vi "myRIOminiVoiceCommand.vi"() -> ()   [LabVIEW 2019]
uses:
  VoiceCommandState.ctl
  <vilib>/myRIO/Common/Instrument Driver Framework/myRIO v1.0/UART/vis/myRIO v1.0 Close UART.vi
  <vilib>/myRIO/Common/Instrument Driver Framework/Utilities/vis/FPGA Ref Manager.vi
  <vilib>/myRIO/Common/Instrument Driver Framework/myRIO v1.0/myRIO v1.0 Reset FPGA.vi
  <vilib>/myRIO/Common/Instrument Driver Framework/myRIO v1.0/IRQ/vis/myRIO v1.0 IRQ Info FGV.vi
  <vilib>/myRIO/Common/Instrument Driver Framework/myRIO v1.0/IRQ/vis/myRIO v1.0 Timer IRQ Info FGV.vi
  <vilib>/myRIO/Common/Instrument Driver Framework/myRIO v1.0/IRQ/vis/myRIO v1.0 ISR Agent.vi
  <vilib>/myRIO/Instrument Drivers/Utilities/vis/Reset Index.vi
  <vilib>/myRIO/Common/Instrument Driver Framework/myRIO v1.0/Resource Manager/vis/myRIO v1.0 Block Write Resource Manager.vi
  Simple Queue Message/Simple Queue Message.lvlib
  <vilib>/myRIO/Instrument Drivers/Utilities/Utilities.lvlib
  Downloads/DFRobot_ASR_myRIO_Lib_ProgramProject/DFRROBOT_ASR_myRIO_Lib/DFRobot_ASR_myRIO.lvlib
panel:
  out "Result out":i32
  out "output array":dbl[][](array[numeric])
  out "heard":i32
  out "distance":i32
  out "command":i32
  out "Correct Key?":bool
  out "Battery (Volts)":dbl format="%.1f"
  out "State":T1
  in  "Stop Button":bool
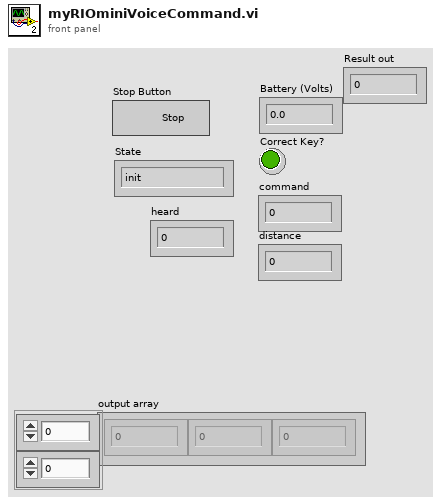
[diagram p1: front panel]
types:
  T1 = typedef "VoiceCommandState.ctl" = enum16{"init", "command", "quantity", "finish", "err"}
  T2 = typedef "miniRef.ctl" = cluster{"Custom FPGA Reference":refnum<k20>, "error out":errorcluster}
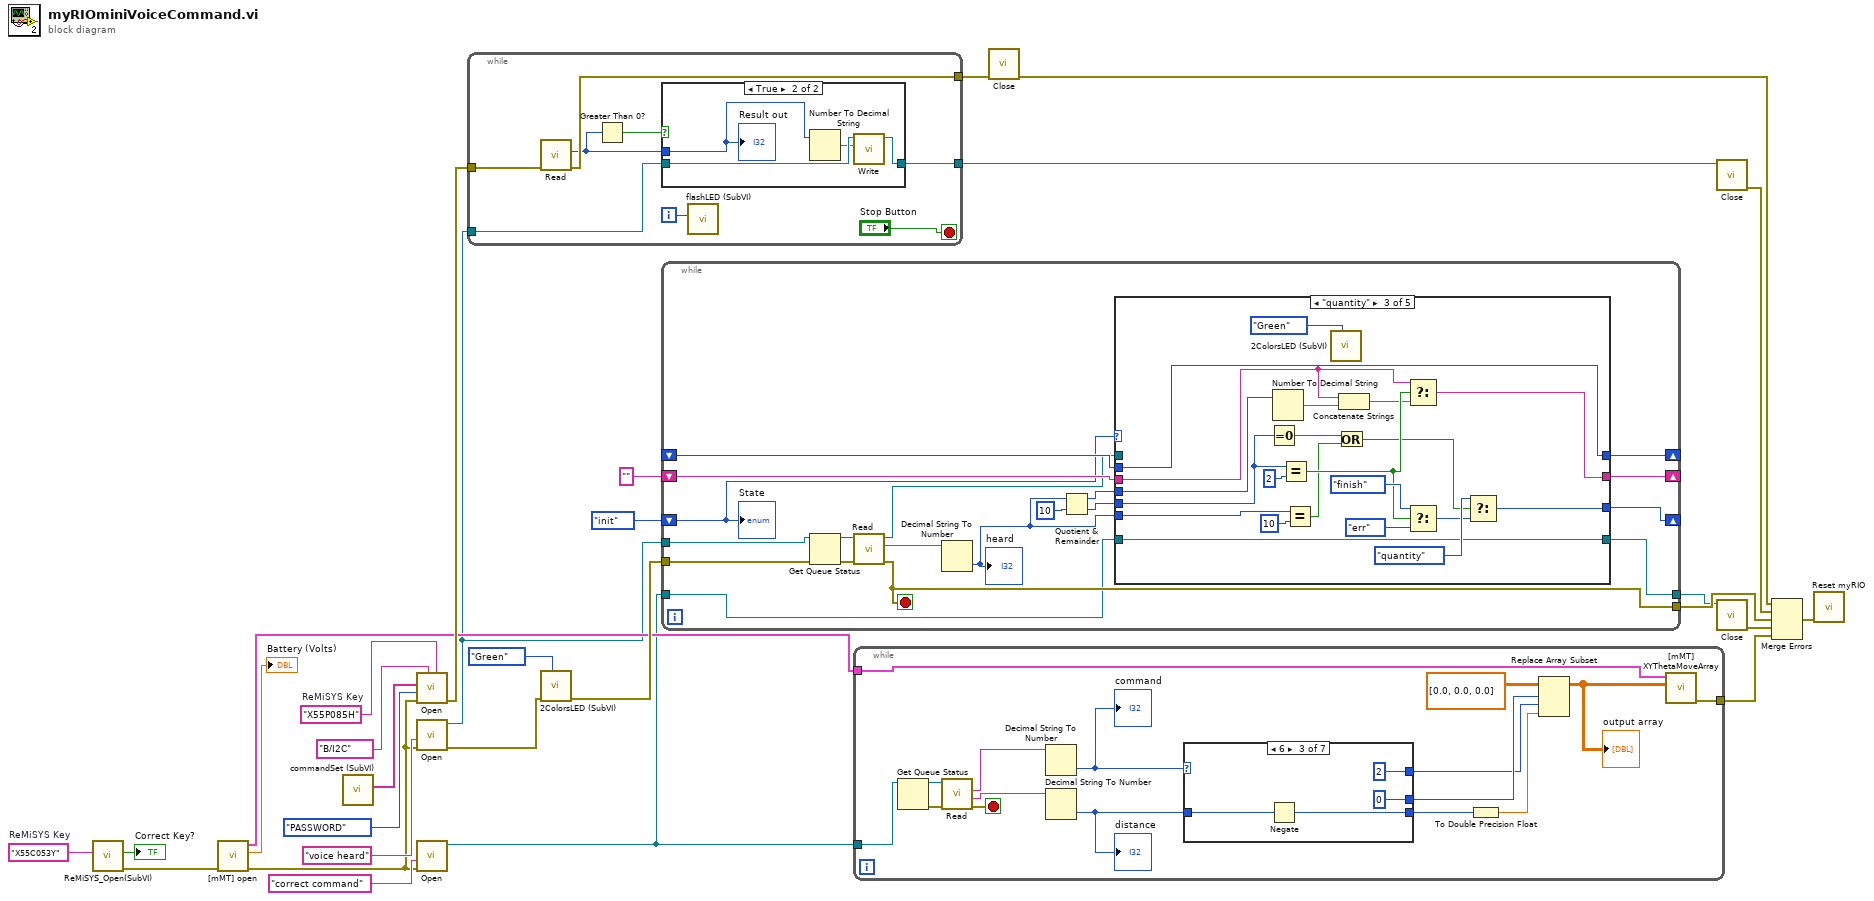
[diagram p0: block diagram]
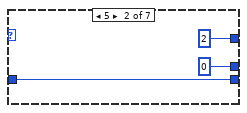
[diagram p3: hidden frame]
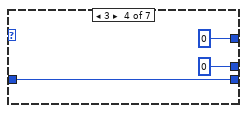
[diagram p4: hidden frame]
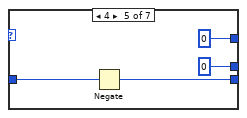
[diagram p5: hidden frame]
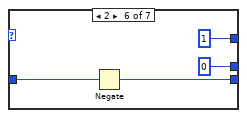
[diagram p6: hidden frame]
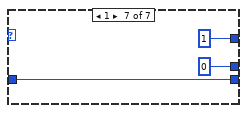
[diagram p7: hidden frame]
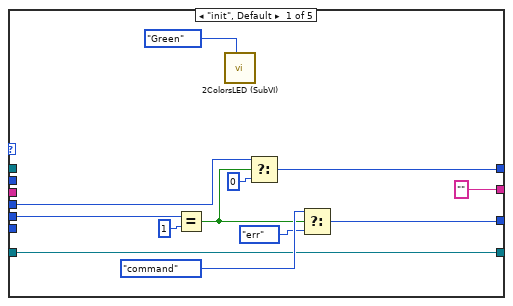
[diagram p8: hidden frame]
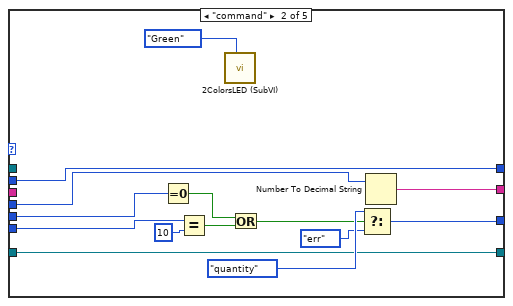
[diagram p9: hidden frame]
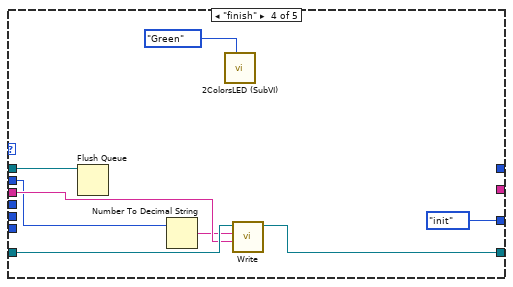
[diagram p10: hidden frame]
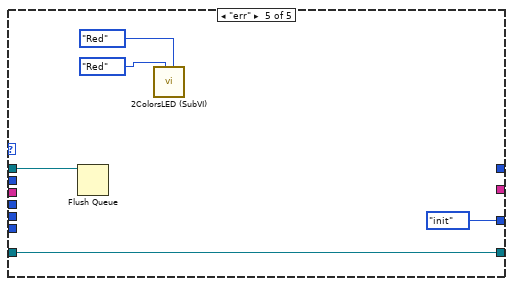
[diagram p11: hidden frame]
diagram:
  w9 = "X55C053Y"  # ReMiSYS Key
  w29 = "X55P085H"  # ReMiSYS Key
  n1 = call <vilib>:"ReMiSYS_Open(SubVI).vi"("ReMiSYS Key"=w9) -> ("error out"=w8:errorcluster, "Correct Key?"=→"Correct Key?":bool)  [unwired: 9 in]
  n2 = call <vilib>:"[mMT] open.vi"("error in"=w8) -> ("error out"=w1:errorcluster, "Battery (Volts)"=→"Battery (Volts)":dbl, "miniOut"=w7:T2)  [unwired: 8 in]
  n3 = call "commandSet (SubVI).vi"() -> ("CommandSet"=w19:string[])  [unwired: 11 in]
  n4 = call "Open.vi"("ReMiSYS Key"=w29, "Channel Name"=tag "B/I2C", "error in (no error)"=w1, "eMode"=enum16{"LOOP", "PASSWORD", "BUTTON"}."PASSWORD", "Command"=w19) -> ("error out"=w28:errorcluster)  [unwired: 6 in]
  n5 = call "Open.vi"("error in (no error)"=w1, "name (unnamed)"="voice heard") -> ("error out"=w15:errorcluster, "queue out"=w2:refnum<queue>)  [unwired: 8 in]
  n6 = call "Open.vi"("error in (no error)"=w1, "name (unnamed)"="correct command") -> ("queue out"=w3:refnum<queue>)  [unwired: 8 in, 1 out]
  n7 = while {
    tunnel: w28 -> [w37]
    tunnel: [w36] -> w25
    tunnel: w2 -> [w34]
    tunnel: [w33] -> w23
    i -> [w30]
    stop <- "Stop Button" stop-if-true
    n8 = call "Read.vi"("error in (no error)"=w37) -> ("error out"=w36:errorcluster, "Result out"=w32:i32)  [unwired: 9 in]
    n9 = Greater Than 0?(x=w32) -> (x > 0?=w31:bool)
    n10 = case shown="True" w31 {
      tunnel: w34 -> [w38 w42]
      tunnel: [w38 w41] -> w33
      tunnel: w32 -> [_ w40]
      frame False {
      }
      frame True {
        n11 = Number To Decimal String(number=w40) -> (decimal integer string=w39:string)  [unwired: 1 in]
        n12 = call "Write.vi"("state"=w39, "queue"=w42) -> ("queue out"=w41:refnum<queue>)  [unwired: 8 in, 1 out]
        "Result out" <- w40
      }
    }
    n13 = call "flashLED (SubVI).vi"("i"=w30) -> ()  [unwired: 11 in]
  }
  n14 = call "2ColorsLED (SubVI).vi"("Color"=enum16{"Green", "Red", "Dimm"}."Green", "error in (no error)"=w15) -> ("error out"=w14:errorcluster)  [unwired: 9 in]
  n15 = while {
    tunnel: w2 -> [w51]
    shift-right: [w60] -> _
    shift-left: VoiceCommandState."init" -> [w47]
    shift-right: [w57] -> _
    shift-left: "" -> [w56]
    shift-right: [w54] -> _
    shift-left: _ -> [w53]
    tunnel: [w48] -> w16
    tunnel: w14 -> [w45]
    tunnel: w3 -> [w44]
    tunnel: [w43] -> w11
    stop <- w48 stop-if-true
    n16 = Get Queue Status(queue=w51, error in (no error)=w45) -> (queue out=w50:refnum<queue>, error out=w49:errorcluster)  [unwired: 1 in, 6 out]
    n17 = call "Read.vi"("error in (no error)"=w49, "queue"=w50) -> ("error out"=w48:errorcluster, "state"=w61:string, "queue out"=w52:refnum<queue>)  [unwired: 6 in, 1 out]
    n18 = Decimal String To Number(string=w61) -> (number=w46:i32)  [unwired: 2 in, 1 out]
    "heard" <- w46
    n19 = Quotient & Remainder(x=w46, y=10) -> (x-y*floor(x/y)=w55:i32, floor(x/y)=w58:i32)
    n20 = case shown="\"quantity\"" w47 {
      tunnel: [w70 w87 w100 VoiceCommandState."init" VoiceCommandState."init"] -> w60
      tunnel: w58 -> [w69 w82 w106 _ _]
      tunnel: ["" w84 w96 _ _] -> w57
      tunnel: w56 -> [_ _ w98 w112 _]
      tunnel: [w66 w83 w101 _ _] -> w54
      tunnel: w55 -> [w67 w81 w88 _ _]
      tunnel: w53 -> [_ w83 w101 w109 _]
      tunnel: w52 -> [_ _ _ w115 w121]
      tunnel: w46 -> [_ w79 w90 _ _]
      tunnel: w44 -> [w62 w74 w94 w113 w117]
      tunnel: [w62 w74 w94 w111 w117] -> w43
      frame "init", Default {
        n21 = Equal?(x=w69, y=1) -> (x = y?=w68:bool)
        n22 = call "2ColorsLED (SubVI).vi"("Color"=enum16{"Green", "Red", "Dimm"}."Green") -> ()  [unwired: 10 in, 1 out]
        n23 = Select(t=w67, s=w68, f=0) -> (s? t:f=w66:i32)
        n24 = Select(t=VoiceCommandState."command", s=w68, f=VoiceCommandState."err") -> (s? t:f=w70:T1)
      }
      frame "command" {
        n25 = Equal To 0?(x=w82) -> (x = 0?=w80:bool)
        n26 = Equal?(x=w79, y=10) -> (x = y?=w77:bool)
        n27 = call "2ColorsLED (SubVI).vi"("Color"=enum16{"Green", "Red", "Dimm"}."Green") -> ()  [unwired: 10 in, 1 out]
        n28 = Or(x=w80, y=w77) -> (x .or. y?=w76:bool)
        n29 = Select(t=VoiceCommandState."quantity", s=w76, f=VoiceCommandState."err") -> (s? t:f=w87:T1)
        n30 = Number To Decimal String(number=w81) -> (decimal integer string=w84:string)  [unwired: 1 in]
      }
      frame "quantity" {
        n31 = Equal To 0?(x=w106) -> (x = 0?=w91:bool)
        n32 = Number To Decimal String(number=w88) -> (decimal integer string=w108:string)  [unwired: 1 in]
        n33 = Equal?(x=w106, y=2) -> (x = y?=w99:bool)
        n34 = Equal?(x=w90, y=10) -> (x = y?=w92:bool)
        n35 = call "2ColorsLED (SubVI).vi"("Color"=enum16{"Green", "Red", "Dimm"}."Green") -> ()  [unwired: 10 in, 1 out]
        n36 = Or(x=w91, y=w92) -> (x .or. y?=w89:bool)
        n37 = Concatenate Strings(w98, w108) -> (w97:string)
        n38 = Select(t=w98, s=w99, f=w97) -> (s? t:f=w96:string)
        n39 = Select(t=VoiceCommandState."finish", s=w99, f=VoiceCommandState."err") -> (s? t:f=w103:T1)
        n40 = Select(t=VoiceCommandState."quantity", s=w89, f=w103) -> (s? t:f=w100:T1)
      }
      frame "finish" {
        n41 = Flush Queue(queue=w115) -> ()  [unwired: 1 in, 3 out]
        n42 = Number To Decimal String(number=w109) -> (decimal integer string=w110:string)  [unwired: 1 in]
        n43 = call "2ColorsLED (SubVI).vi"("Color"=enum16{"Green", "Red", "Dimm"}."Green") -> ()  [unwired: 10 in, 1 out]
        n44 = call "Write.vi"("payload"=w112, "state"=w110, "queue"=w113) -> ("queue out"=w111:refnum<queue>)  [unwired: 7 in, 1 out]
      }
      frame "err" {
        n45 = Flush Queue(queue=w121) -> ()  [unwired: 1 in, 3 out]
        n46 = call "2ColorsLED (SubVI).vi"("Color 2"=enum16{"Green", "Red", "Dimm"}."Red", "Color"=enum16{"Green", "Red", "Dimm"}."Red") -> ()  [unwired: 9 in, 1 out]
      }
    }
    "State" <- w47
  }
  n47 = while {
    tunnel: w3 -> [w134]
    tunnel: w7 -> [w133]
    tunnel: [w122] -> w4
    stop <- w135 stop-if-true
    n48 = Get Queue Status(queue=w134) -> (queue out=w137:refnum<queue>, error out=w136:errorcluster)  [unwired: 2 in, 6 out]
    n49 = call "Read.vi"("error in (no error)"=w136, "queue"=w137) -> ("error out"=w135:errorcluster, "payload"=w131:string, "state"=w132:string)  [unwired: 6 in, 1 out]
    n50 = Decimal String To Number(string=w132) -> (number=w130:i32)  [unwired: 2 in, 1 out]
    "command" <- w130
    n51 = Decimal String To Number(string=w131) -> (number=w125:i32)  [unwired: 2 in, 1 out]
    "distance" <- w125
    n52 = case shown="6" w130 {
      tunnel: [_ 0 ("index") 0 ("index") 0 ("index") 0 ("index") 0 ("index") 0 ("index")] -> w128
      tunnel: [_ 2 ("index") 2 ("index") 0 ("index") 0 ("index") 1 ("index") 1 ("index")] -> w127
      tunnel: [_ w138 w141 w147 w148 w154 w156] -> w126
      tunnel: w125 -> [_ w138 w142 w147 w149 w155 w156]
      frame 0, Default {
      }
      frame 5 {
      }
      frame 6 {
        n53 = Negate(x=w142) -> (-x=w141:i32)
      }
      frame 3 {
      }
      frame 4 {
        n54 = Negate(x=w149) -> (-x=w148:i32)
      }
      frame 2 {
        n55 = Negate(x=w155) -> (-x=w154:i32)
      }
      frame 1 {
      }
    }
    n56 = To Double Precision Float(number=w126) -> (double precision float=w124:dbl)
    n57 = Replace Array Subset(array=dbl[][] [[0.0, 0.0, 0.0]] ("XYZ"), new element=w124, index (row)=w128, index (col)=w127) -> (w123:dbl[][])
    "output array" <- w123
    n58 = call <vilib>:"[mMT] XYThetaMoveArray.vi"("XYZ"=w123, "miniOut"=w133) -> ("error out"=w122:errorcluster)  [unwired: 8 in, 1 out]
  }
  n59 = call "Close.vi"("error in (no error)"=w25) -> ("error out"=w18:errorcluster)  [unwired: 10 in]
  n60 = call "Close.vi"("queue out"=w23) -> ("error out"=w17:errorcluster)  [unwired: 10 in]
  n61 = call "Close.vi"("queue out"=w11) -> ("error out"=w10:errorcluster)  [unwired: 10 in]
  n62 = Merge Errors(w18, w17, w16, w10, w4) -> (w21:errorcluster)
  n63 = call <vilib>:"Reset myRIO.vi"("error in (no error)"=w21) -> ()  [unwired: 10 in, 1 out]
